vi "Calc_RPM.vi"(11 "Distance Type":enum16{"SONAR", "VISION", "BOTH"}(ring)=enum."VISION") -> (1 "Calculation_Ready":bool, 2 "In_Range":bool, 3 "Suggested Speed":dbl)   [LabVIEW 2015]
uses:
  <vilib>/Analysis/baseanly.llb/Mean (DBL).vi
  Robot Global Data.vi
  <vilib>/Analysis/NI_AALPro.lvlib
  <vilib>/Analysis/NI_AALBase.lvlib
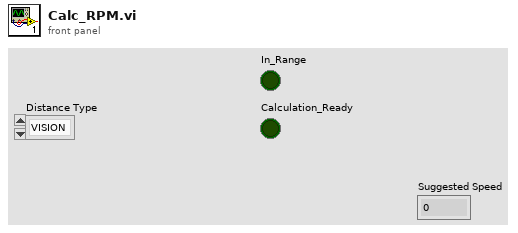
[diagram p1: front panel]
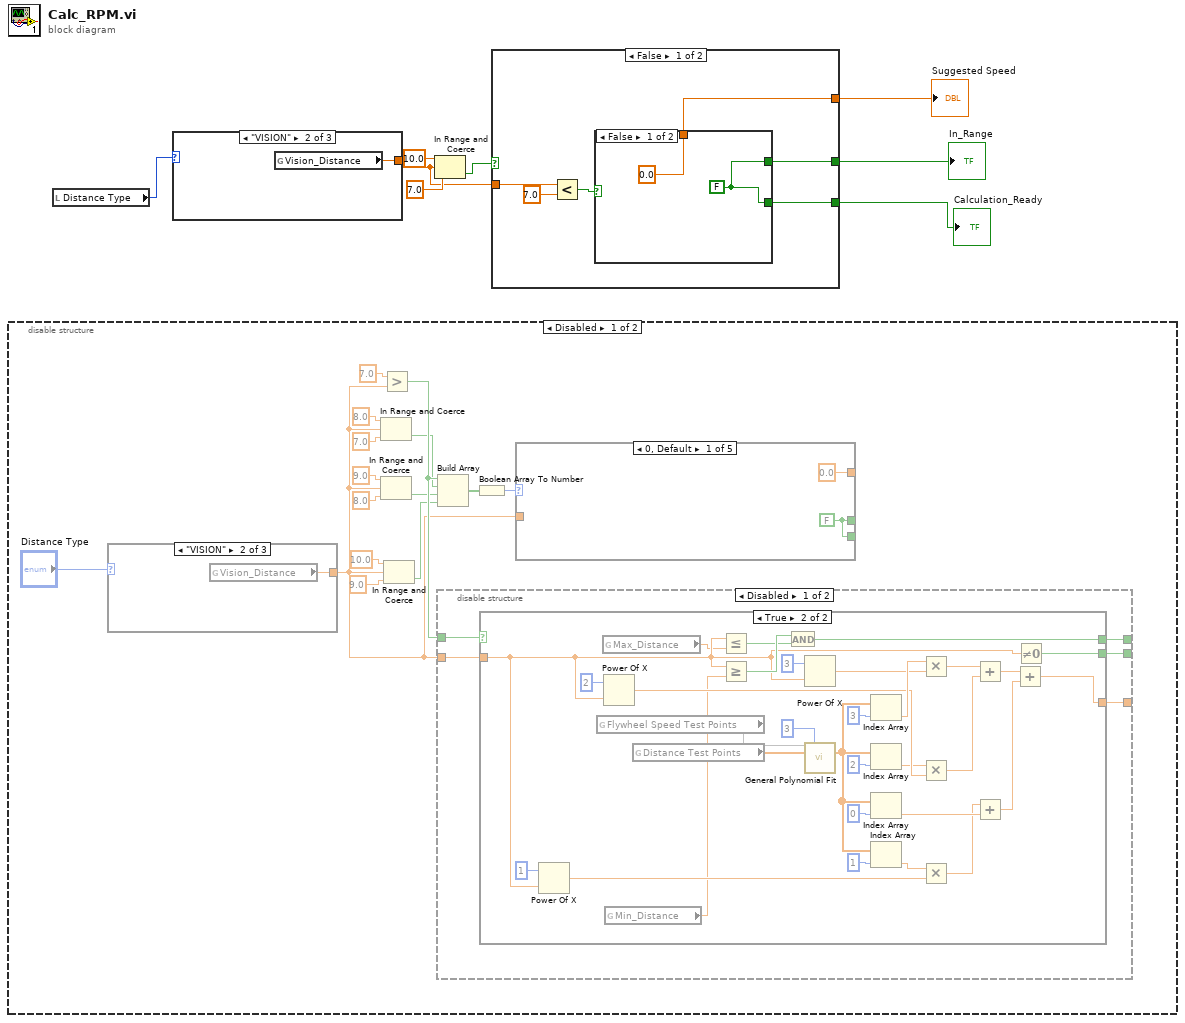
[diagram p0: block diagram]
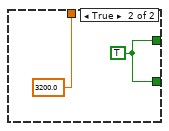
[diagram p2: hidden frame]
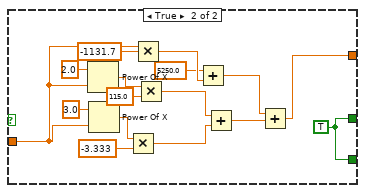
[diagram p3: hidden frame]
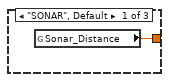
[diagram p4: hidden frame]
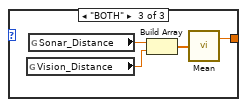
[diagram p5: hidden frame]
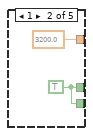
[diagram p6: hidden frame]
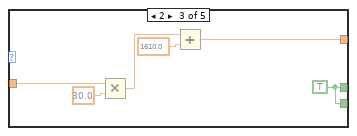
[diagram p7: hidden frame]
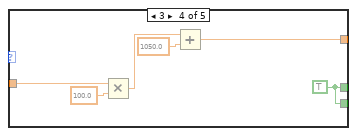
[diagram p8: hidden frame]
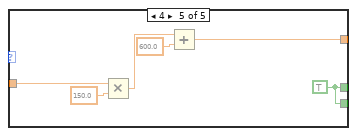
[diagram p9: hidden frame]
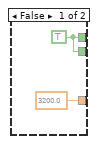
[diagram p10: hidden frame]
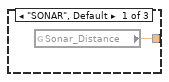
[diagram p12: hidden frame]
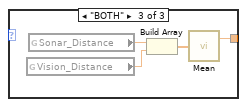
[diagram p13: hidden frame]
diagram:
  n1 = disable-structure shown="Disabled" {
    frame Disabled {
      n2 = case shown="\"VISION\"" "Distance Type" {
        tunnel: [w87 w88 w89] -> w9
        frame "SONAR", Default {
          n3 = global read "Robot Global Data.vi" "Sonar_Distance"() -> (w87:dbl)
        }
        frame "VISION" {
          n4 = global read "Robot Global Data.vi" "Vision_Distance"() -> (w88:dbl)
        }
        frame "BOTH" {
          n5 = global read "Robot Global Data.vi" "Vision_Distance"() -> (w92:dbl)
          n6 = global read "Robot Global Data.vi" "Sonar_Distance"() -> (w91:dbl)
          n7 = Build Array(w91, w92) -> (w90:dbl[])
          n8 = call-poly <vilib>:"Mean.vi"("X"=w90) -> ("mean"=w89:dbl)  [unwired: 1 out]
        }
      }
      n9 = In Range and Coerce(upper limit=8.0, x=w9, lower limit=7.0) -> (In Range?=w23:bool)  [unwired: 1 out]
      n10 = In Range and Coerce(upper limit=9.0, x=w9, lower limit=8.0) -> (In Range?=w18:bool)  [unwired: 1 out]
      n11 = Greater?(x=7.0, y=w9) -> (0:w24:bool)
      n12 = In Range and Coerce(upper limit=10.0, x=w9, lower limit=9.0) -> (In Range?=w15:bool)  [unwired: 1 out]
      n13 = Build Array(w24, w23, w18, w15) -> (w14:bool[])
      n14 = disable-structure shown="Disabled" {
        disable-tunnel: [w53 _] -> _
        disable-tunnel: [w52 _] -> _
        disable-tunnel: [w51 _] -> _
        disable-tunnel: w24 -> [w50 _]
        disable-tunnel: w9 -> [w49 _]
        frame Disabled {
          n15 = case shown="True" w50 {
            tunnel: w49 -> [_ w63]
            tunnel: [3200.0 w58] -> w53
            tunnel: [w54 w57] -> w52
            tunnel: [w54 w56] -> w51
            frame False {
              w54 = TRUE
            }
            frame True {
              n16 = Power Of X(1:w63, 2:1) -> (0:w75:dbl)
              n17 = global read "Robot Global Data.vi" "Flywheel Speed Test Points"() -> (w59)
              n18 = global read "Robot Global Data.vi" "Max_Distance"() -> (w62:dbl)
              n19 = Power Of X(1:w63, 2:2) -> (0:w79:dbl)
              n20 = global read "Robot Global Data.vi" "Min_Distance"() -> (w61:dbl)
              n21 = global read "Robot Global Data.vi" "Distance Test Points"() -> (w60:dbl[])
              n22 = Less Or Equal?(x=w63, y=w62) -> (x <= y?=w64:bool)
              n23 = Greater Or Equal?(x=w63, y=w61) -> (x >= y?=w65:bool)
              n24 = And(x=w65, y=w64) -> (x .and. y?=w56:bool)
              n25 = Power Of X(1:w63, 2:3) -> (0:w80:dbl)
              n26 = call <vilib>:"General Polynomial Fit.vi"("Y"=w59, "polynomial order"=3, "X"=w60) -> ("Polynomial Coefficients"=w77:dbl[])  [unwired: 9 in, 3 out]
              n27 = Index Array(array=w77, index=3) -> (element=w81:dbl)
              n28 = Index Array(array=w77, index=2) -> (element=w78:dbl)
              n29 = Index Array(array=w77, index=0) -> (element=w72:dbl)
              n30 = Index Array(array=w77, index=1) -> (element=w76:dbl)
              n31 = Multiply(x=w81, y=w80) -> (x*y=w74:dbl)
              n32 = Multiply(x=w78, y=w79) -> (x*y=w73:dbl)
              n33 = Multiply(x=w76, y=w75) -> (x*y=w71:dbl)
              n34 = Add(x=w74, y=w73) -> (x+y=w70:dbl)
              n35 = Add(x=w71, y=w72) -> (x+y=w69:dbl)
              n36 = Add(x=w70, y=w69) -> (x+y=w58:dbl)
              n37 = Not Equal To 0?(x=w63) -> (x != 0?=w57:bool)
            }
          }
        }
        frame Enabled {
        }
      }
      n38 = Boolean Array To Number(Boolean array=w14) -> (number=w13:u32)
      n39 = case shown="0, Default" w13 {
        tunnel: [w28 w29 w31 w42 w43] -> w12
        tunnel: [0.0 3200.0 w32 w37 w46] -> w11
        tunnel: w9 -> [_ _ w36 w41 w48]
        tunnel: [w28 w29 w31 w42 w43] -> w10
        frame 0, Default {
          w28 = FALSE
        }
        frame 1 {
          w29 = TRUE
        }
        frame 2 {
          w31 = TRUE
          n40 = Multiply(x=w36, y=30.0) -> (x*y=w34:dbl)
          n41 = Add(x=w34, y=1610.0) -> (x+y=w32:dbl)
        }
        frame 3 {
          w42 = TRUE
          n42 = Multiply(x=w41, y=100.0) -> (x*y=w39:dbl)
          n43 = Add(x=w39, y=1050.0) -> (x+y=w37:dbl)
        }
        frame 4 {
          w43 = TRUE
          n44 = Multiply(x=w48, y=150.0) -> (x*y=w47:dbl)
          n45 = Add(x=w47, y=600.0) -> (x+y=w46:dbl)
        }
      }
    }
    frame Enabled {
    }
  }
  n46 = local read "Distance Type"() -> (w8:enum16{"SONAR", "VISION", "BOTH"})
  n47 = case shown="\"VISION\"" w8 {
    tunnel: [w93 w94 w95] -> w2
    frame "SONAR", Default {
      n48 = global read "Robot Global Data.vi" "Sonar_Distance"() -> (w93:dbl)
    }
    frame "VISION" {
      n49 = global read "Robot Global Data.vi" "Vision_Distance"() -> (w94:dbl)
    }
    frame "BOTH" {
      n50 = global read "Robot Global Data.vi" "Vision_Distance"() -> (w98:dbl)
      n51 = global read "Robot Global Data.vi" "Sonar_Distance"() -> (w97:dbl)
      n52 = Build Array(w97, w98) -> (w96:dbl[])
      n53 = call-poly <vilib>:"Mean.vi"("X"=w96) -> ("mean"=w95:dbl)  [unwired: 1 out]
    }
  }
  n54 = In Range and Coerce(upper limit=10.0, x=w2, lower limit=7.0) -> (In Range?=w7:bool)  [unwired: 1 out]
  n55 = case shown="False" w7 {
    tunnel: [w101 w124] -> w4
    tunnel: [w100 w124] -> w3
    tunnel: w2 -> [w104 w117]
    tunnel: [w99 w111] -> w1
    frame False {
      n56 = Less?(x=w104, y=7.0) -> (x < y?=w102:bool)
      n57 = case shown="False" w102 {
        tunnel: [w106 w108] -> w101
        tunnel: [w106 w108] -> w100
        tunnel: [0.0 3200.0] -> w99
        frame False {
          w106 = FALSE
        }
        frame True {
          w108 = TRUE
        }
      }
    }
    frame True {
      w124 = TRUE
      n58 = Power Of X(1:w117, 2:2.0 ("y")) -> (0:w119:dbl)
      n59 = Power Of X(1:w117, 2:3.0 ("y")) -> (0:w122:dbl)
      n60 = Multiply(x=w122, y=-3.333) -> (x*y=w114:dbl)
      n61 = Multiply(x=w117, y=-1131.7) -> (x*y=w110:dbl)
      n62 = Multiply(x=w119, y=115.0) -> (x*y=w115:dbl)
      n63 = Add(x=5250.0, y=w110) -> (x+y=w113:dbl)
      n64 = Add(x=w115, y=w114) -> (x+y=w112:dbl)
      n65 = Add(x=w113, y=w112) -> (x+y=w111:dbl)
    }
  }
  "In_Range" <- w4
  "Suggested Speed" <- w1
  "Calculation_Ready" <- w3
